vi "DT_Cal Cos Angle_Core.vi"(6 "y3":dbl, 7 "x1":dbl, 8 "y2":dbl, 9 "y1":dbl, 10 "x3":dbl, 11 "x2":dbl) -> (3 "angle":dbl)   [LabVIEW 2020, in "NI_AAL_Geometry.lvlib"]
uses:
  <vilib>/Analysis/NI_AAL_Geometry.lvlib
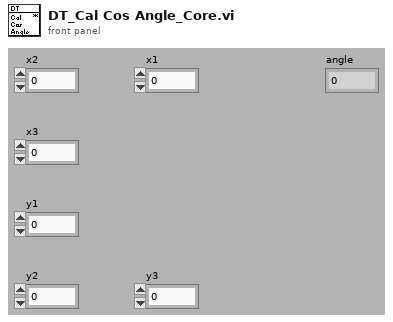
[diagram p1: front panel]
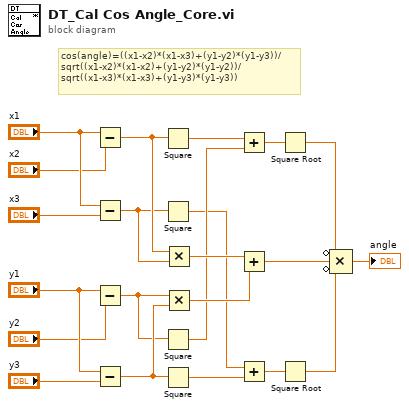
[diagram p0: block diagram]
diagram:
  # "cos(angle)=((x1-x2)*(x1-x3)+(y1-y2)*(y1-y3))/\nsqrt((x1-x2)*(x1-x2)+(y1-y2)*(y1-y2))/\nsqrt((x1-x3)*(x1-x3)+(y1-y3)*(y1-y3))"
  n1 = Subtract(x="x1", y="x2") -> (x-y=w22:dbl)
  n2 = Subtract(x="x1", y="x3") -> (x-y=w15:dbl)
  n3 = Subtract(x="y1", y="y2") -> (x-y=w14:dbl)
  n4 = Subtract(x="y1", y="y3") -> (x-y=w21:dbl)
  n5 = Square(x=w22) -> (x^2=w11:dbl)
  n6 = Square(x=w15) -> (x^2=w9:dbl)
  n7 = Square(x=w14) -> (x^2=w10:dbl)
  n8 = Square(x=w21) -> (x^2=w8:dbl)
  n9 = Multiply(x=w22, y=w15) -> (x*y=w13:dbl)
  n10 = Multiply(x=w14, y=w21) -> (x*y=w12:dbl)
  n11 = Add(x=w11, y=w10) -> (x+y=w20:dbl)
  n12 = Add(x=w13, y=w12) -> (x+y=w18:dbl)
  n13 = Add(x=w9, y=w8) -> (x+y=w19:dbl)
  n14 = Square Root(x=w20) -> (sqrt(x)=w17:dbl)
  n15 = Square Root(x=w19) -> (sqrt(x)=w16:dbl)
  n16 = Compound Arithmetic op=MULTIPLY(invert w17, w18, invert w16) -> (→"angle":dbl)
